vi "RND320PowerSupply.vi"(6 "raw":string="GMOD", 7 "Command":T1(ring)=enum."GetActualUI", 8 "error in (no error)":errorcluster, 9 "Ampere":dbl, 10 "Volt in":dbl, 11 "VISA resource name":refnum<visa-resource-name>) -> (0 "error out":errorcluster, 1 "Ampere out":dbl, 2 "Volt out":dbl, 3 "VISA resource name out":refnum<visa-resource-name>, 4 "String":string)   [LabVIEW 2011]
uses:
  <vilib>/Instr/_visa.llb/VISA Flush IO Buffer Mask.ctl
  <vilib>/Instr/_visa.llb/VISA Configure Serial Port (Instr).vi
panel:
  out "raw Bytes at Serial Port":u32
  # "9600,8N1\ncr?\n*IDN?"
  # "reaction time ~1s"
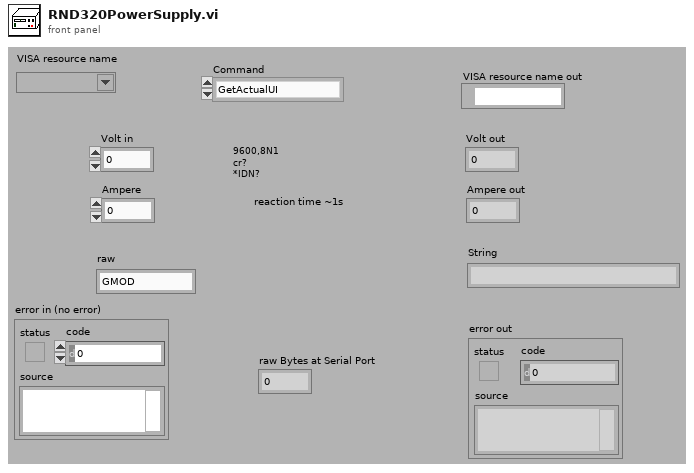
[diagram p1: front panel]
types:
  T1 = enum16{"No Operation", "GetActualUI", "GetSetpointsUI", "SetUI", "SetU", "SetI", "OutputOff", "OutputOn", "GetLimitU", "GetLimitI", "SetLimitU", "SetLimitI", "GetUI-fromVersion", "RawCommand"}
  T2 = typedef "VISA Flush IO Buffer Mask.ctl" = u16
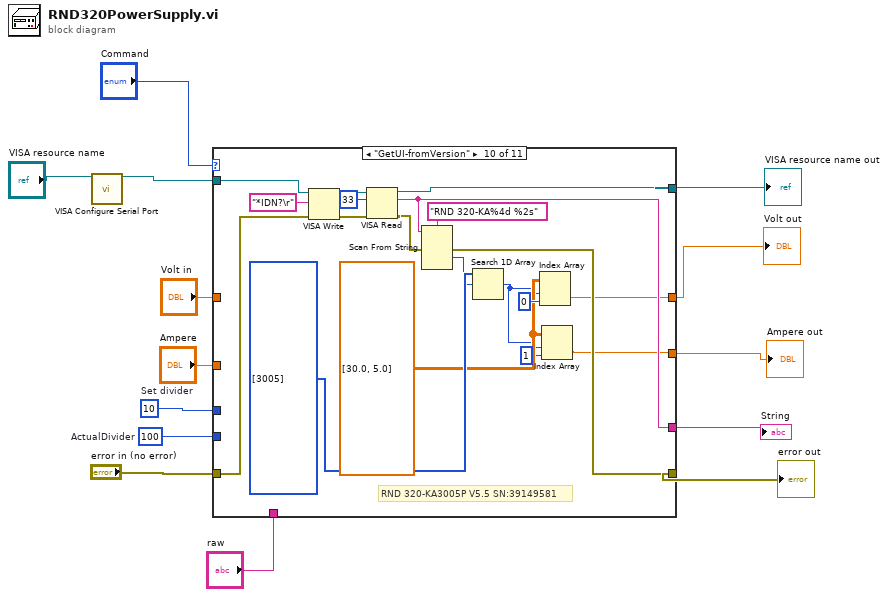
[diagram p0: block diagram]
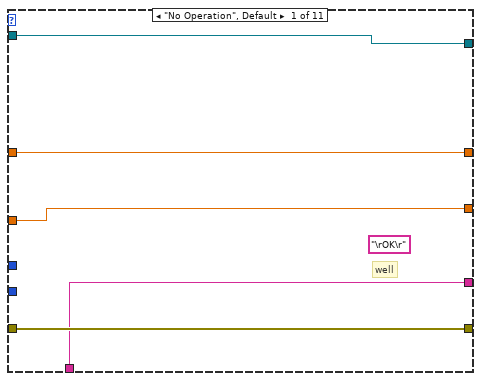
[diagram p2: hidden frame]
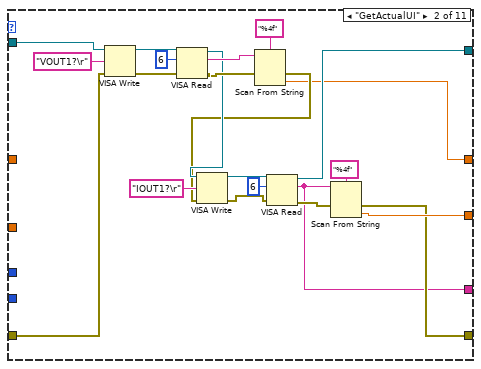
[diagram p3: hidden frame]
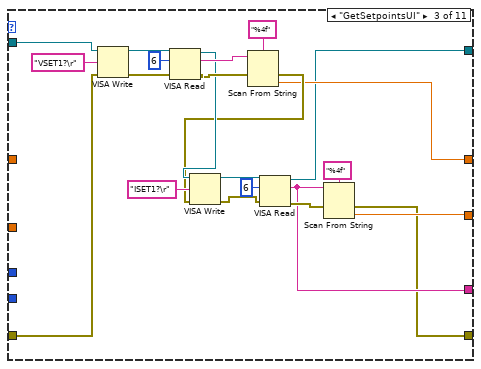
[diagram p4: hidden frame]
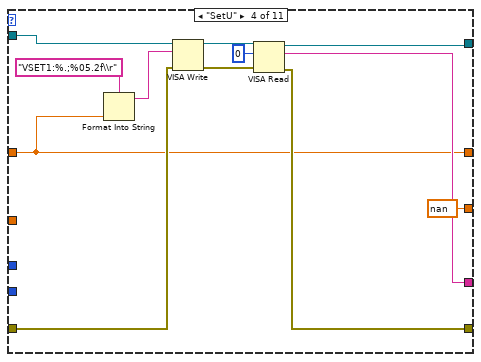
[diagram p5: hidden frame]
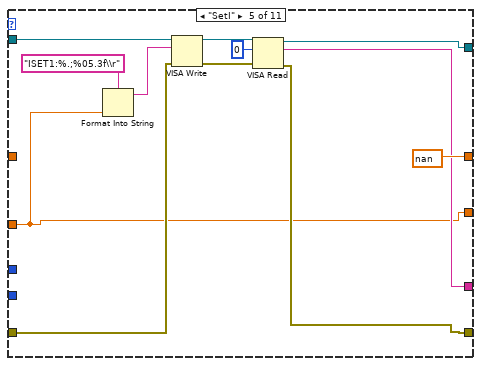
[diagram p6: hidden frame]
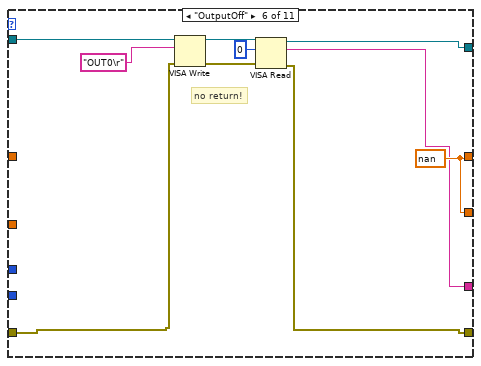
[diagram p7: hidden frame]
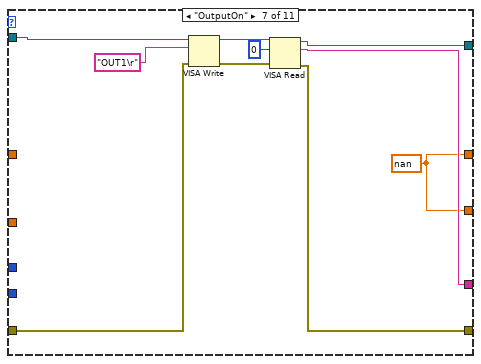
[diagram p8: hidden frame]
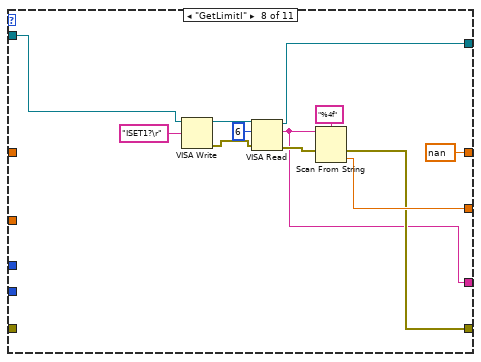
[diagram p9: hidden frame]
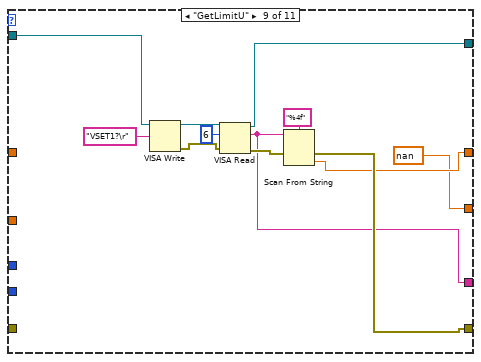
[diagram p10: hidden frame]
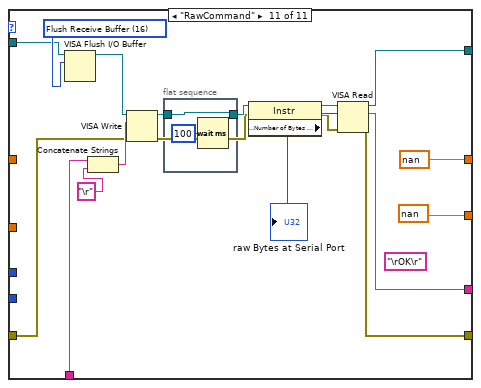
[diagram p11: hidden frame]
diagram:
  w2 = 100  # ActualDivider
  w3 = 10  # Set divider
  n1 = call-poly "VISA Configure Serial Port"("VISA resource name"="VISA resource name") -> ("VISA resource name out"=w4:refnum<visa-resource-name>)  [unwired: 5 in, 9 out]
  n2 = case shown="\"GetUI-fromVersion\"" "Command" {
    tunnel: w4 -> [w19 w41 w48 w75 w82 w94 w103 w109 w125 w145 w161]
    tunnel: [w19 w27 w43 w71 w81 w93 w100 w112 w120 w144 w155] -> w13
    tunnel: "error in (no error)" -> [w18 w40 w47 w70 w77 w92 w102 _ _ w143 w163]
    tunnel: [w18 w21 w42 w68 w78 w91 w101 w111 w124 w140 w151] -> w1
    tunnel: [w15 w20 w46 w66 w79 w88 w99 w110 w123 w142 w154] -> w10
    tunnel: "raw" -> [w15 _ _ _ _ _ _ _ _ _ w166]
    tunnel: "Ampere" -> [w16 _ _ _ w76 _ _ _ _ _ _]
    tunnel: "Volt in" -> [w17 _ _ w64 _ _ _ _ _ _ _]
    tunnel: [w16 w22 w45 nan ("Ampere") w76 w90 w98 w113 nan ("Volt in") w132 nan ("Ampere")] -> w6
    tunnel: [w17 w23 w44 w64 nan ("Ampere") w90 w98 nan ("Volt in") w122 w133 nan ("Volt in")] -> w5
    tunnel: w3 -> [_ _ _ _ _ _ _ _ _ _ _]
    tunnel: w2 -> [_ _ _ _ _ _ _ _ _ _ _]
    frame "No Operation", Default {
      (unwired) "\rOK\r"
      # "well"
    }
    frame "GetActualUI" {
      n3 = VISA Write(VISA resource name=w41, write buffer="VOUT1?\r", error in (no error)=w40) -> (VISA resource name out=w37:refnum<visa-resource-name>, error out=w39:errorcluster)  [unwired: 1 out]
      n4 = VISA Read(VISA resource name=w37, byte count=u32 6, error in (no error)=w39) -> (VISA resource name out=w28:refnum<visa-resource-name>, read buffer=w35:string, error out=w33:errorcluster)  [unwired: 1 out]
      n5 = Scan From String(format string="%4f", input string=w35, error in=w33) -> (error out=w26:errorcluster, output 1=w23:dbl)  [unwired: 1 in, 3 out]
      n6 = VISA Write(VISA resource name=w28, write buffer="IOUT1?\r", error in (no error)=w26) -> (VISA resource name out=w31:refnum<visa-resource-name>, error out=w25:errorcluster)  [unwired: 1 out]
      n7 = VISA Read(VISA resource name=w31, byte count=u32 6, error in (no error)=w25) -> (VISA resource name out=w27:refnum<visa-resource-name>, read buffer=w20:string, error out=w24:errorcluster)  [unwired: 1 out]
      n8 = Scan From String(format string="%4f", input string=w20, error in=w24) -> (error out=w21:errorcluster, output 1=w22:dbl)  [unwired: 1 in, 3 out]
    }
    frame "GetSetpointsUI" {
      n9 = VISA Write(VISA resource name=w48, write buffer="VSET1?\r", error in (no error)=w47) -> (VISA resource name out=w61:refnum<visa-resource-name>, error out=w63:errorcluster)  [unwired: 1 out]
      n10 = VISA Read(VISA resource name=w61, byte count=u32 6, error in (no error)=w63) -> (VISA resource name out=w52:refnum<visa-resource-name>, read buffer=w59:string, error out=w57:errorcluster)  [unwired: 1 out]
      n11 = Scan From String(format string="%4f", input string=w59, error in=w57) -> (error out=w51:errorcluster, output 1=w44:dbl)  [unwired: 1 in, 3 out]
      n12 = VISA Write(VISA resource name=w52, write buffer="ISET1?\r", error in (no error)=w51) -> (VISA resource name out=w55:refnum<visa-resource-name>, error out=w50:errorcluster)  [unwired: 1 out]
      n13 = VISA Read(VISA resource name=w55, byte count=u32 6, error in (no error)=w50) -> (VISA resource name out=w43:refnum<visa-resource-name>, read buffer=w46:string, error out=w49:errorcluster)  [unwired: 1 out]
      n14 = Scan From String(format string="%4f", input string=w46, error in=w49) -> (error out=w42:errorcluster, output 1=w45:dbl)  [unwired: 1 in, 3 out]
    }
    frame "SetU" {
      n15 = Format Into String(format string="VSET1:%.;%05.2f\\r", w64) -> (resulting string=w73:string)  [unwired: 2 in, 1 out]
      n16 = VISA Write(VISA resource name=w75, write buffer=w73, error in (no error)=w70) -> (VISA resource name out=w72:refnum<visa-resource-name>, error out=w69:errorcluster)  [unwired: 1 out]
      n17 = VISA Read(VISA resource name=w72, byte count=u32 0, error in (no error)=w69) -> (VISA resource name out=w71:refnum<visa-resource-name>, read buffer=w66:string, error out=w68:errorcluster)  [unwired: 1 out]
    }
    frame "SetI" {
      n18 = Format Into String(format string="ISET1:%.;%05.3f\\r", w76) -> (resulting string=w84:string)  [unwired: 2 in, 1 out]
      n19 = VISA Write(VISA resource name=w82, write buffer=w84, error in (no error)=w77) -> (VISA resource name out=w85:refnum<visa-resource-name>, error out=w86:errorcluster)  [unwired: 1 out]
      n20 = VISA Read(VISA resource name=w85, byte count=u32 0, error in (no error)=w86) -> (VISA resource name out=w81:refnum<visa-resource-name>, read buffer=w79:string, error out=w78:errorcluster)  [unwired: 1 out]
    }
    frame "OutputOff" {
      w90 = nan ("Ampere")
      # "no return!"
      n21 = VISA Write(VISA resource name=w94, write buffer="OUT0\r" ("format string"), error in (no error)=w92) -> (VISA resource name out=w97:refnum<visa-resource-name>, error out=w96:errorcluster)  [unwired: 1 out]
      n22 = VISA Read(VISA resource name=w97, byte count=u32 0, error in (no error)=w96) -> (VISA resource name out=w93:refnum<visa-resource-name>, read buffer=w88:string, error out=w91:errorcluster)  [unwired: 1 out]
    }
    frame "OutputOn" {
      w98 = nan ("Ampere")
      n23 = VISA Write(VISA resource name=w103, write buffer="OUT1\r" ("format string"), error in (no error)=w102) -> (VISA resource name out=w107:refnum<visa-resource-name>, error out=w106:errorcluster)  [unwired: 1 out]
      n24 = VISA Read(VISA resource name=w107, byte count=u32 0, error in (no error)=w106) -> (VISA resource name out=w100:refnum<visa-resource-name>, read buffer=w99:string, error out=w101:errorcluster)  [unwired: 1 out]
    }
    frame "GetLimitI" {
      n25 = VISA Write(VISA resource name=w109, write buffer="ISET1?\r") -> (VISA resource name out=w118:refnum<visa-resource-name>, error out=w115:errorcluster)  [unwired: 1 in, 1 out]
      n26 = VISA Read(VISA resource name=w118, byte count=u32 6, error in (no error)=w115) -> (VISA resource name out=w112:refnum<visa-resource-name>, read buffer=w110:string, error out=w114:errorcluster)  [unwired: 1 out]
      n27 = Scan From String(format string="%4f", input string=w110, error in=w114) -> (error out=w111:errorcluster, output 1=w113:dbl)  [unwired: 1 in, 3 out]
    }
    frame "GetLimitU" {
      n28 = VISA Write(VISA resource name=w125, write buffer="VSET1?\r") -> (VISA resource name out=w130:refnum<visa-resource-name>, error out=w127:errorcluster)  [unwired: 1 in, 1 out]
      n29 = VISA Read(VISA resource name=w130, byte count=u32 6, error in (no error)=w127) -> (VISA resource name out=w120:refnum<visa-resource-name>, read buffer=w123:string, error out=w126:errorcluster)  [unwired: 1 out]
      n30 = Scan From String(format string="%4f", input string=w123, error in=w126) -> (error out=w124:errorcluster, output 1=w122:dbl)  [unwired: 1 in, 3 out]
    }
    frame "GetUI-fromVersion" {
      w137 = sgl[][] [[30.0, 5.0]]
      # "RND 320-KA3005P V5.5 SN:39149581"
      n31 = VISA Write(VISA resource name=w145, write buffer="*IDN?\r", error in (no error)=w143) -> (VISA resource name out=w148:refnum<visa-resource-name>, error out=w146:errorcluster)  [unwired: 1 out]
      n32 = VISA Read(VISA resource name=w148, byte count=u32 33, error in (no error)=w146) -> (VISA resource name out=w144:refnum<visa-resource-name>, read buffer=w142:string, error out=w141:errorcluster)  [unwired: 1 out]
      n33 = Scan From String(format string="RND 320-KA%4d %2s", input string=w142, error in=w141) -> (error out=w140:errorcluster, output 1=w134:i32)  [unwired: 1 in, 5 out]
      n34 = Search 1D Array(1D array=i32[] [3005], element=w134) -> (index of element=w135:i32)  [unwired: 1 out]
      n35 = Index Array(array=w137, index (row)=w135, index (col)=0 ("disabled index (col)")) -> (element=w133:sgl)
      n36 = Index Array(array=w137, index (row)=w135, index (col)=1 ("disabled index (col)")) -> (element=w132:sgl)
    }
    frame "RawCommand" {
      w162 = T2 16 items=["Flush Receive Buffer"=16, "Write Transmit Buffer to Device"=32, "Flush Receive Buffer (No I/O)"=64, "Flush Transmit Buffer"=128] ("Mask")
      (unwired) "\rOK\r"
      n37 = VISA Flush I/O Buffer(VISA resource name=w161, mask (16)=w162) -> (VISA resource name out=w160:refnum<visa-resource-name>)  [unwired: 1 in, 1 out]
      n38 = Concatenate Strings(w166, "\r" ("write buffer")) -> (w164:string)
      n39 = VISA Write(VISA resource name=w160, write buffer=w164, error in (no error)=w163) -> (VISA resource name out=w159:refnum<visa-resource-name>, error out=w157:errorcluster)  [unwired: 1 out]
      n40 = flat-sequence {
        tunnel: w159 -> [w169]
        tunnel: [w169] -> w158
        frame #0 {
          n41 = Wait (ms)(milliseconds to wait=u32 100) -> ()  [unwired: 1 out]
        }
      }
      n42 = property class="Instr"(reference=w158, error in=w157) -> (reference out=w168:refnum<visa-resource-name>, error out=w156:errorcluster, "Serial Settings:Number of Bytes at Serial Port"=w167:u32)
      "raw Bytes at Serial Port" <- w167
      n43 = VISA Read(VISA resource name=w168, byte count=w167, error in (no error)=w156) -> (VISA resource name out=w155:refnum<visa-resource-name>, read buffer=w154:string, error out=w151:errorcluster)  [unwired: 1 out]
    }
  }
  "Volt out" <- w5
  "VISA resource name out" <- w13
  "error out" <- w1
  "Ampere out" <- w6
  "String" <- w10
